vi "New Waveform Buffer.vi"(8 "error in (no error)":errorcluster, 10 "Buffer Duration":dbl, 11 "Buffer Data Type":T1) -> (0 "error out":errorcluster, 3 "Waveform Buffer out":refnum<class "Waveform Buffer.lvclass">)   [LabVIEW 2015, in "Waveform Buffer.lvclass"]
uses:
  Waveform Buffer.lvclass
  Buffer Data Type.ctl
  DBL Waveform Buffer/DBL Waveform Buffer.lvclass
  CDB Waveform Buffer/CDB Waveform Buffer.lvclass
  Waveform Buffer.lvclass/Waveform Buffer.ctl
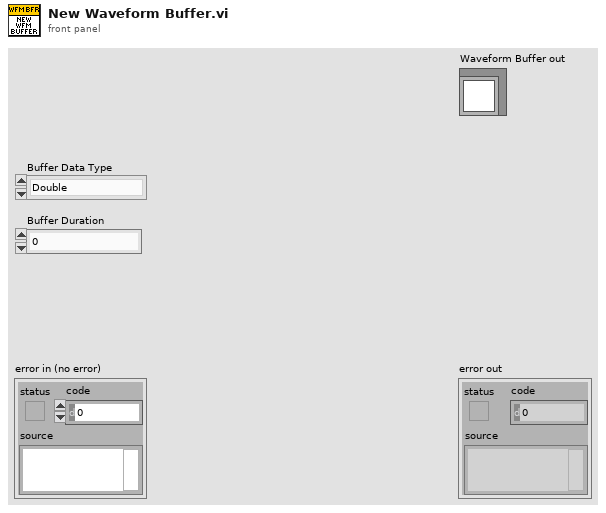
[diagram p1: front panel]
types:
  T1 = typedef "Waveform Buffer.lvclass/Buffer Data Type.ctl" = enum16{"Double", "ComplexDouble"}
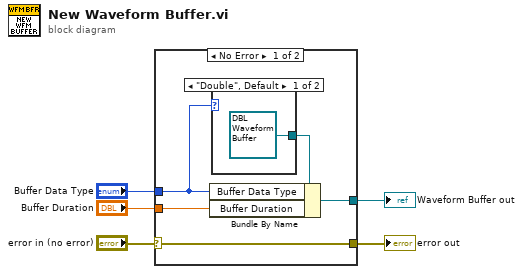
[diagram p0: block diagram]
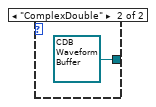
[diagram p2: hidden frame]
diagram:
  n1 = case shown="No Error" "error in (no error)" {
    selector: "error in (no error)" -> [w7 w13]
    tunnel: [w7 w13] -> w4
    tunnel: [w6 _] -> w3
    tunnel: "Buffer Data Type" -> [w9 _]
    tunnel: "Buffer Duration" -> [w8 _]
    frame No Error {
      n2 = case shown="\"Double\", Default" w9 {
        tunnel: [refnum<class "DBL Waveform Buffer.lvclass"> refnum ("Waveform Data Logger Engine.lvlib:DBL Waveform Buffer.lvclass") refnum<class "CDB Waveform Buffer.lvclass"> refnum ("Waveform Data Logger Engine.lvlib:CDB Waveform Buffer.lvclass")] -> w10
        frame "Double", Default {
        }
        frame "ComplexDouble" {
        }
      }
      n3 = Bundle By Name(cluster=w10, "Buffer Data Type"=w9, "Buffer Duration"=w8) -> (w6:refnum<class "Waveform Buffer.lvclass">)
    }
    frame Error {
    }
  }
  "error out" <- w4
  "Waveform Buffer out" <- w3
